vi "Rawdata_Metadata_Generator.vi"() -> ()   [LabVIEW 2020]
uses:
  ctl/Image_Configuration.ctl
  ctl/Image_RAW_Bayer_Pattern.ctl
  ctl/Image_EBD_Config.ctl
panel:
  in  "Camera Type":enum16{"Side", "Front"}(ring)
  in  "stop":bool
  out "Progress":dbl(slide) scale=0.0..100.0
  out "error out":errorcluster
  in  "Output File Path":path
  in  "Timestamp Type":enum16{"Base", "Base +/- Rand(Delta T)"}(ring)=enum."Base +/- Rand(Delta T)"
  in  "Delta T (ns)":u64=1000000
  in  "Base Relative Time (ns)":u64=33000000
  in  "Num of Frames to generate":u32=5000
  in  "T0":timestamp
  in  "Bayer Pattern":T1=enum."RGGB (GRBG)"
  in  "Image Data Type":u8=44 format="%x"
  in  "Image Configuration":T2={"Width"=1920, "Height"=1080}
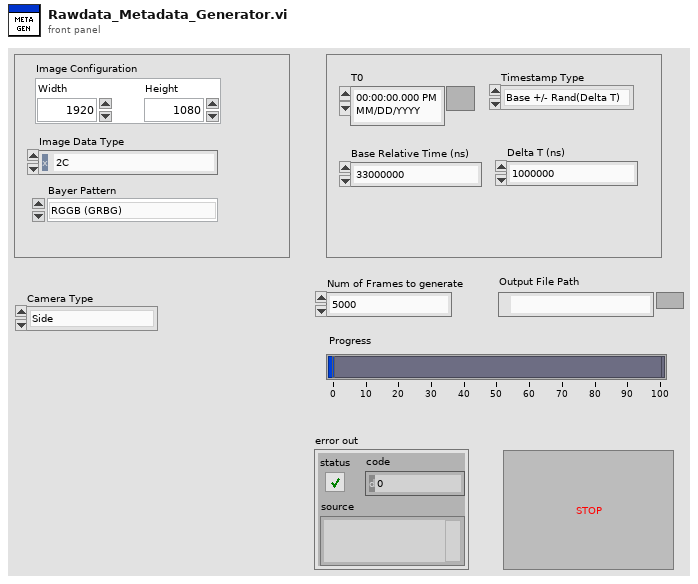
[diagram p1: front panel]
types:
  T1 = typedef "Image_RAW_Bayer_Pattern.ctl" = enum16{"GBRG (BGGR)", "GRBG (RGGB)", "BGGR (GBRG)", "RGGB (GRBG)", "CRBC (RCCB)"}
  T2 = typedef "Image_Configuration.ctl" = cluster{"Width":i32, "Height":i32}
  T3 = enum16{"open", "replace", "create", "open or create", "replace or create", "replace or create with confirmation"}
  T4 = typedef "Image_Data_Config.ctl" = cluster{"Lines of Image Data":u16, "Bytes per Even Line":u16, "Bytes per Odd Line":u16, "Image Data Type":u8, "Total Image Data Block Size":u32, "Image Data Block Offset":u32}
  T5 = enum16{"big-endian, network order", "native, host order", "little-endian"}
  T6 = typedef "Image_EBD_Config.ctl" = cluster{"Lines of Pre-EBD Data":u16, "Lines of Post-EBD Data":u16, "Total EBD Block Size":u32, "Pre-EBD Block Offset ":u32, "Post-EBD Block Offset ":u32}
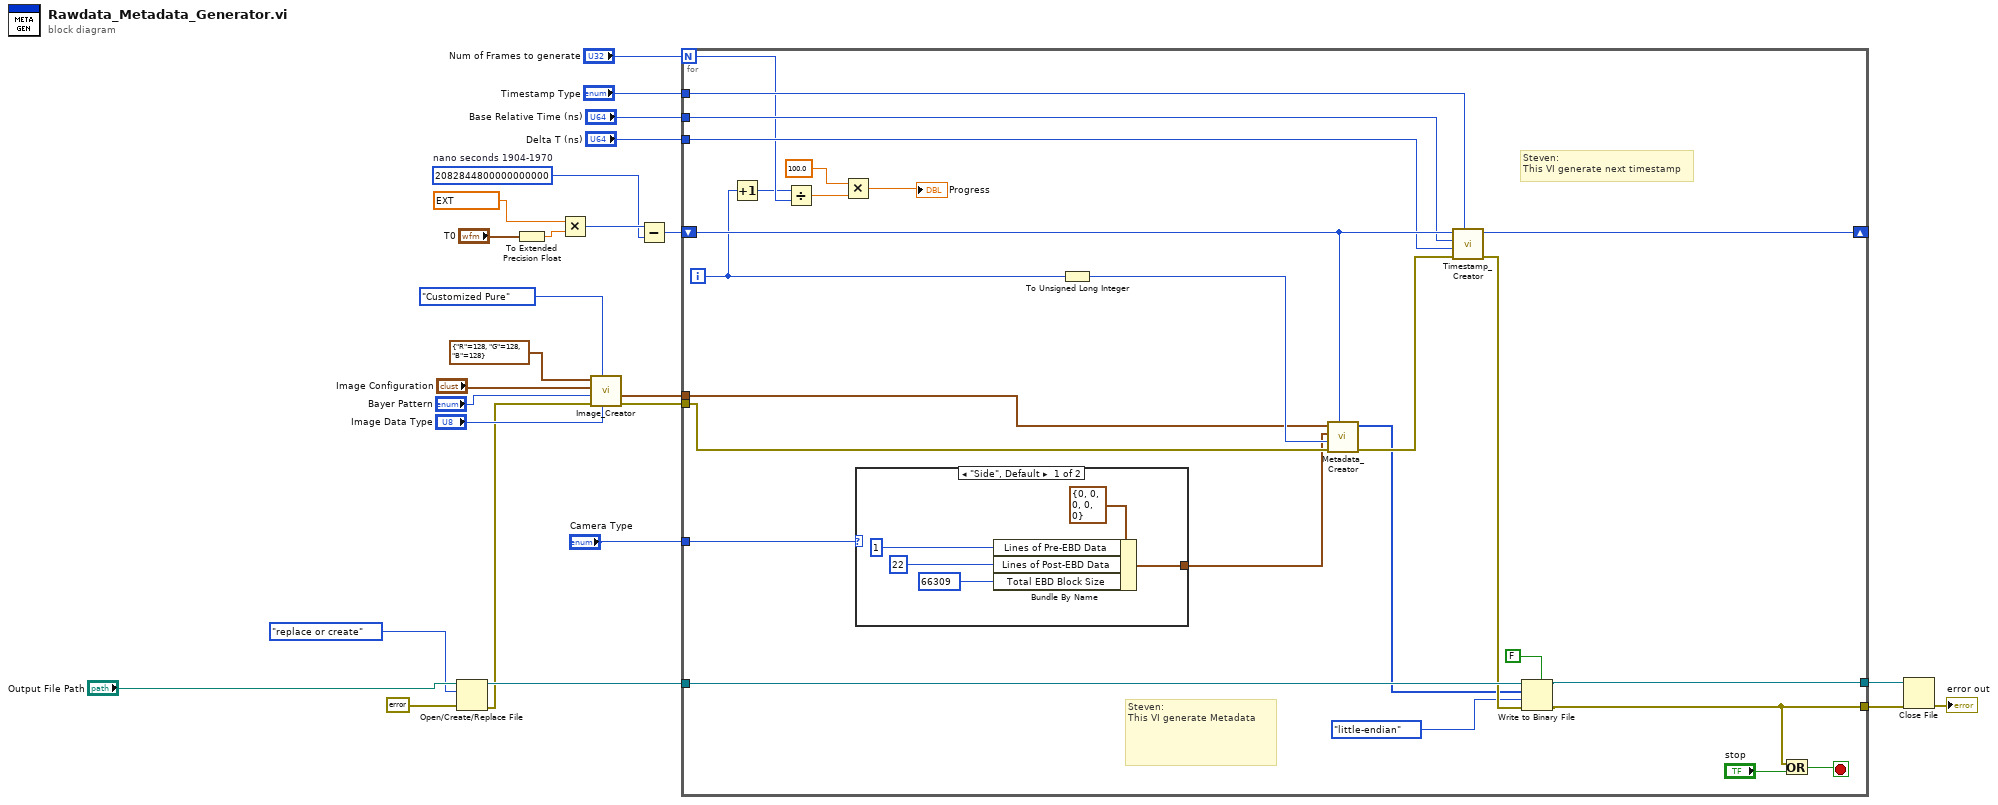
[diagram p0: block diagram]
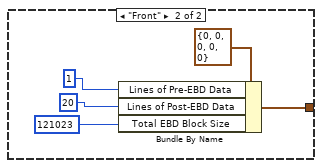
[diagram p2: hidden frame]
diagram:
  w21 = u64 2082844800000000000  # nano seconds 1904-1970
  n1 = Open/Create/Replace File(file path (use dialog)="Output File Path", error in=errorcluster {"status"=FALSE, "code"=0, "source"=""} ("error in (no error)"), operation (0:open)=T3."replace or create") -> (refnum out=w13:refnum<file>, error out=w4:errorcluster)  [unwired: 3 in, 1 out]
  n2 = To Extended Precision Float(1:"T0") -> (0:w22:ext)
  n3 = Multiply(x=ext 1000000000.0, y=w22) -> (x*y=w23:u64)
  n4 = call "Image_Creator.vi"("Image Data Type"="Image Data Type", "Pattern"=enum16{"24 Color Checker", "Customized Pure"}."Customized Pure", "error in (no error)"=w4, "Bayer Pattern"="Bayer Pattern", "Image Configuration"="Image Configuration", "Pure Color Pattern Parameters"=cluster{"R":u8, "G":u8, "B":u8} {"R"=128, "G"=128, "B"=128}) -> ("error out"=w3:errorcluster, "Image Data Config"=w2:T4)  [unwired: 2 in, 2 out]
  n5 = Subtract(x=w23, y=w21) -> (x-y=w18:u64)
  n6 = for {
    N: "Num of Frames to generate" -> [w39]
    shift-right: [w46] -> _
    shift-left: w18 -> [w50]
    tunnel: "Timestamp Type" -> [w49]
    tunnel: "Base Relative Time (ns)" -> [w48]
    tunnel: "Delta T (ns)" -> [w47]
    tunnel: w13 -> [w45]
    tunnel: [w32] -> w12
    tunnel: [w31] -> w11
    tunnel: w3 -> [w30]
    tunnel: w2 -> [w29]
    tunnel: "Camera Type" -> [w28]
    i -> [w40]
    stop <- w34 stop-if-true
    # "Steven:\nThis VI generate Metadata"
    # "Steven:\nThis VI generate next timestamp"
    n7 = Increment(x=w40) -> (x+1=w33:i32)
    n8 = Divide(x=w33, y=w39) -> (x/y=w38:dbl)
    n9 = Multiply(x=100.0, y=w38) -> (x*y=→"Progress":dbl)
    n10 = case shown="\"Side\", Default" w28 {
      tunnel: [w53 w58] -> w27
      frame "Side", Default {
        n11 = Bundle By Name(cluster=T6 {"Lines of Pre-EBD Data"=0, "Lines of Post-EBD Data"=0, "Total EBD Block Size"=0, "Pre-EBD Block Offset "=0, "Post-EBD Block Offset "=0} ("EBD Config"), "Lines of Pre-EBD Data"=u16 1, "Lines of Post-EBD Data"=u16 22, "Total EBD Block Size"=u32 66309) -> (w53:T6)
      }
      frame "Front" {
        n12 = Bundle By Name(cluster=T6 {"Lines of Pre-EBD Data"=0, "Lines of Post-EBD Data"=0, "Total EBD Block Size"=0, "Pre-EBD Block Offset "=0, "Post-EBD Block Offset "=0} ("EBD Config"), "Lines of Pre-EBD Data"=u16 1, "Lines of Post-EBD Data"=u16 20, "Total EBD Block Size"=u32 121023) -> (w58:T6)
      }
    }
    n13 = To Unsigned Long Integer(number=w40) -> (unsigned 32bit integer=w52:u32)
    n14 = call "Metadata_Creator.vi"("Frame Timestamp"=w50, "error in (no error)"=w30, "Frame Index"=w52, "EBD Config"=w27, "Image Data Config"=w29) -> ("error out"=w51:errorcluster, "Meta Data (U8)"=w43:u8[])  [unwired: 5 in]
    n15 = call "Timestamp_Creator.vi"("Timestamp Type"=w49, "error in (no error)"=w51, "Delta T (ns)"=w47, "Base Relative Time (ns)"=w48, "Previous Time (ns)"=w50) -> ("error out"=w44:errorcluster, "Next Time (ns)"=w46:u64)  [unwired: 5 in]
    n16 = Write to Binary File(file (use dialog)=w45, data=w43, error in=w44, 5:FALSE ("prepend array or string size? (T)"), 9:T5."little-endian" ("byte order (0:big-endian, network order)")) -> (refnum out=w32:refnum<file>, error out=w31:errorcluster)  [unwired: 1 in, 1 out]
    n17 = Or(x=w31, y="stop") -> (x .or. y?=w34:bool)
  }
  n18 = Close File(refnum=w12, error in=w11) -> (error out=→"error out":errorcluster)  [unwired: 1 out]
